vi "Message Nested Object.vi"(8 "error in (no error)":errorcluster, 9 "Message":refnum<class "Message.lvclass">, 10 "Name":string, 11 "Application Controller in":refnum<class "Template Module.lvclass">) -> (0 "error out":errorcluster, 3 "Application Controller out":refnum<class "Template Module.lvclass">)   [LabVIEW 2016, in "Template Module.lvclass"]
uses:
  Template Module.lvclass
  C:/Program Files (x86)/National Instruments/LabVIEW 2016/vi.lib/ActorFramework/Actor/Actor.lvclass
  <vilib>/ActorFramework/Message/Message.lvclass
  <vilib>/ActorFramework/Actor/Actor.lvclass/Actor.ctl
  Template Module Messages/Message Nested Object Msg/Message Nested Object Msg.lvclass/Message Nested Object Msg.ctl
  <vilib>/ActorFramework/Message Enqueuer/Message Enqueuer.lvclass/Message Enqueuer.ctl
  Template Module Messages/Message Nested Object Msg/Message Nested Object Msg.lvclass
  C:/Program Files (x86)/National Instruments/LabVIEW 2016/vi.lib/ActorFramework/Message/Message.lvclass
  <vilib>/ActorFramework/Message Priority Queue/Priority Enqueue.vi
  <vilib>/ActorFramework/Message Enqueuer/Message Enqueuer.lvclass
  <vilib>/ActorFramework/Actor/Actor.lvclass
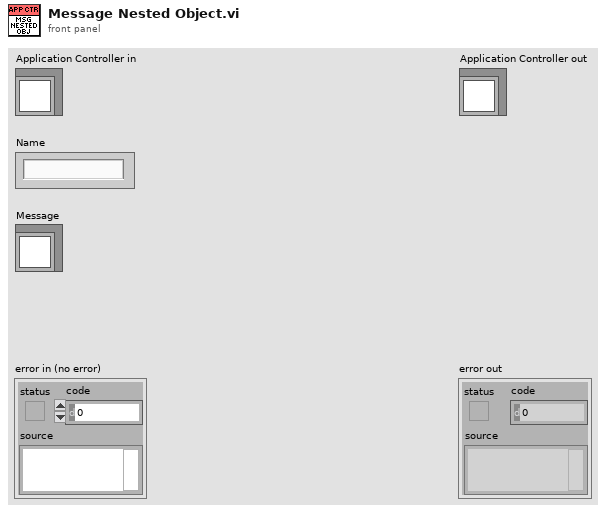
[diagram p1: front panel]
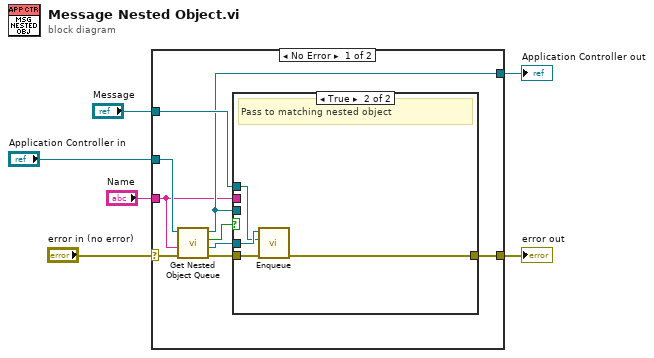
[diagram p0: block diagram]
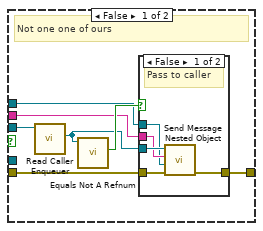
[diagram p2: hidden frame]
diagram:
  n1 = case shown="No Error" "error in (no error)" {
    selector: "error in (no error)" -> [w13 w34]
    tunnel: [w9 w34] -> w5
    tunnel: [w8 w33] -> w3
    tunnel: "Application Controller in" -> [w14 w33]
    tunnel: "Name" -> [w7 _]
    tunnel: "Message" -> [w10 _]
    frame No Error {
      n2 = call-dynamic "Get Nested Object Queue.vi"("error in (no error)"=w13, "Name"=w7, "Measure Object in"=w14) -> ("error out"=w11:errorcluster, "Object Enqueuer"=w12:refnum<class "Message Enqueuer.lvclass">, "Found?"=w15:bool, "Measure Object out"=w8:refnum<class "Template Module.lvclass">)  [unwired: 5 in]
      n3 = case shown="True" w15 {
        tunnel: w12 -> [_ w32]
        tunnel: w11 -> [w20 w31]
        tunnel: w10 -> [w16 w30]
        tunnel: [w19 w29] -> w9
        tunnel: w8 -> [w22 _]
        tunnel: w7 -> [w17 _]
        frame False {
          # "Not one one of ours"
          n4 = call <vilib>:"Read Caller Enqueuer.vi"("Actor"=w22) -> ("Caller Enqueuer"=w18:refnum<class "Message Enqueuer.lvclass">)  [unwired: 10 in]
          n5 = call <vilib>:"Equals Not A Refnum.vi"("Message Enqueuer"=w18) -> ("Not a refnum?"=w21:bool)  [unwired: 10 in]
          n6 = case shown="False" w21 {
            tunnel: w20 -> [w27 w28]
            tunnel: [w26 w28] -> w19
            tunnel: w18 -> [w25 _]
            tunnel: w17 -> [w24 _]
            tunnel: w16 -> [w23 _]
            frame False {
              # "Pass to caller"
              n7 = call "Send Message Nested Object.vi"("error in (no error)"=w27, "Message"=w23, "Name"=w24, "Message Enqueuer"=w25) -> ("error out"=w26:errorcluster)  [unwired: 6 in, 1 out]
            }
            frame True {
            }
          }
        }
        frame True {
          # "Pass to matching nested object"
          n8 = call <vilib>:"Enqueue.vi"("error in (no error)"=w31, "Message"=w30, "Message Enqueuer in"=w32) -> ("error out"=w29:errorcluster)  [unwired: 7 in, 1 out]
        }
      }
    }
    frame Error {
    }
  }
  "error out" <- w5
  "Application Controller out" <- w3
